vi "ddsPhaseArrayConvert.vi"(7 "Pre 3.0 AOM driver version?":bool, 10 "Register":dbl=5.0 min=0.0 max=15.0 step=1.0 format="%#.1f", 11 "Phase Array (degrees)":dbl[](array[numeric])=[0.0] min=0.0 max=360.0 step=0.022 format="%.2g") -> (3 "Characters for FPGA":string="L50000\r\n")   [LabVIEW 2013, in "DDS9954_v2013.lvlib"]
uses:
  DDS9954_v2013.lvlib
  dataToAscii_16bit.vi
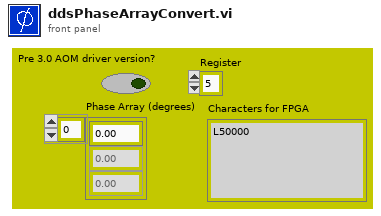
[diagram p1: front panel]
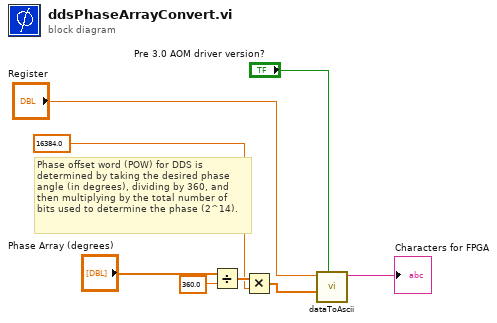
[diagram p0: block diagram]
diagram:
  # "Phase offset word (POW) for DDS is\ndetermined by taking the desired phase \nangle (in degrees), dividing by 360, and \nthen multiplying by the total number of \nbits used to determine the phase (2^14)."
  n1 = Divide(x="Phase Array (degrees)", y=360.0) -> (x/y=w7:dbl[])
  n2 = Multiply(x=w7, y=16384.0) -> (x*y=w2:dbl[])
  n3 = call-poly "dataToAscii.vi"("Pre 3.0 AOM driver version?"="Pre 3.0 AOM driver version?", "Input Data"=w2, "Register"="Register") -> ("Characters to FPGA"=→"Characters for FPGA":string)  [unwired: 8 in]
